vi "Verify Select All.vi"(0 "TreeControl in":refnum<vi>, 5 "Measurement Tags":string[](array[string]), 11 "error in (no error)":errorcluster) -> (4 "TreeControl out":refnum<vi>, 6 "Select":bool, 8 "Deselect":bool, 15 "error out":errorcluster)   [LabVIEW 2021, in "Converter.lvlib"]
uses:
  Converter.lvlib
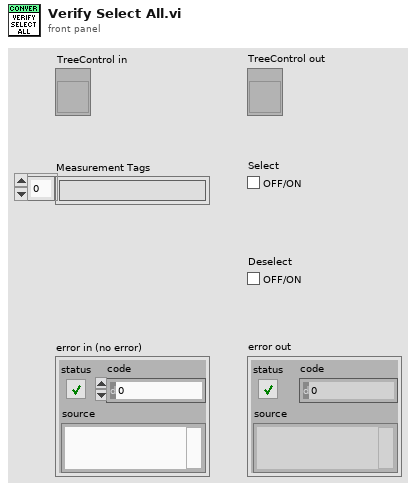
[diagram p1: front panel]
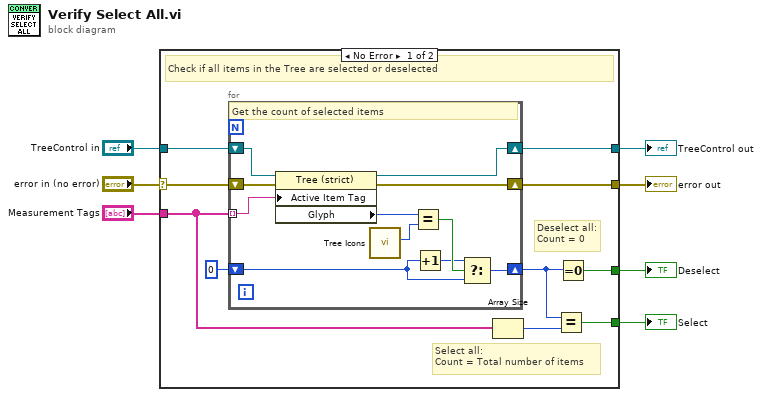
[diagram p0: block diagram]
diagram:
  n1 = case shown="No Error" "error in (no error)" {
    selector: "error in (no error)" -> [w15 w30]
    tunnel: "Measurement Tags" -> [w17 _]
    tunnel: "TreeControl in" -> [w14 w29]
    tunnel: [w11 _] -> w4
    tunnel: [w10 _] -> w3
    tunnel: [w9 w30] -> w2
    tunnel: [w8 w29] -> w1
    frame No Error {
      # "Select all:\nCount = Total number of items"
      # "Deselect all:\nCount = 0"
      # "Check if all items in the Tree are selected or deselected"
      n2 = for {
        shift-right: [w20] -> w9
        shift-left: w15 -> [w28]
        tunnel: w17 -> [w27] mode=indexing
        shift-right: [w21] -> w13
        shift-left: 0 -> [w22]
        shift-right: [w18] -> w8
        shift-left: w14 -> [w19]
        # "Get the count of selected items"
        n3 = property on="Property Node" class="Tree (strict)"(reference=w19, error in=w28, "Active Item Tag"=w27) -> (reference out=w18:refnum<vi>, error out=w20:errorcluster, "Glyph"=w26:i32)
        n4 = call "Tree Icons.vi"() -> ("Selected"=w25:i32)  [unwired: 6 in, 1 out]
        n5 = Equal?(x=w26, y=w25) -> (x = y?=w24:bool)
        n6 = Increment(x=w22) -> (x+1=w23:i32)
        n7 = Select(t=w23, s=w24, f=w22) -> (s? t:f=w21:i32)
      }
      n8 = Array Size(array=w17) -> (size(s)=w12:i32)
      n9 = Equal?(x=w13, y=w12) -> (x = y?=w10:bool)
      n10 = Equal To 0?(x=w13) -> (x = 0?=w11:bool)
    }
    frame Error {
      # "Pass"
    }
  }
  "error out" <- w2
  "Deselect" <- w4
  "Select" <- w3
  "TreeControl out" <- w1
